vi "LV SciSDK REGISTER FILE SET REGISTER.vi"(8 "error in (no error)":errorcluster, 9 "Register File Handle In":T2, 10 "Register Name":string, 11 "Value":i32) -> (0 "error out":errorcluster, 1 "Register File Handle Out":T2)   [LabVIEW 2021, in "SciSDK_Labview.lvlib"]
uses:
  SciSDK_Labview.lvlib
panel:
  out "NI Error Code":i32
  out "Board Handle Out":T1
  in  "Board Handle In":T1
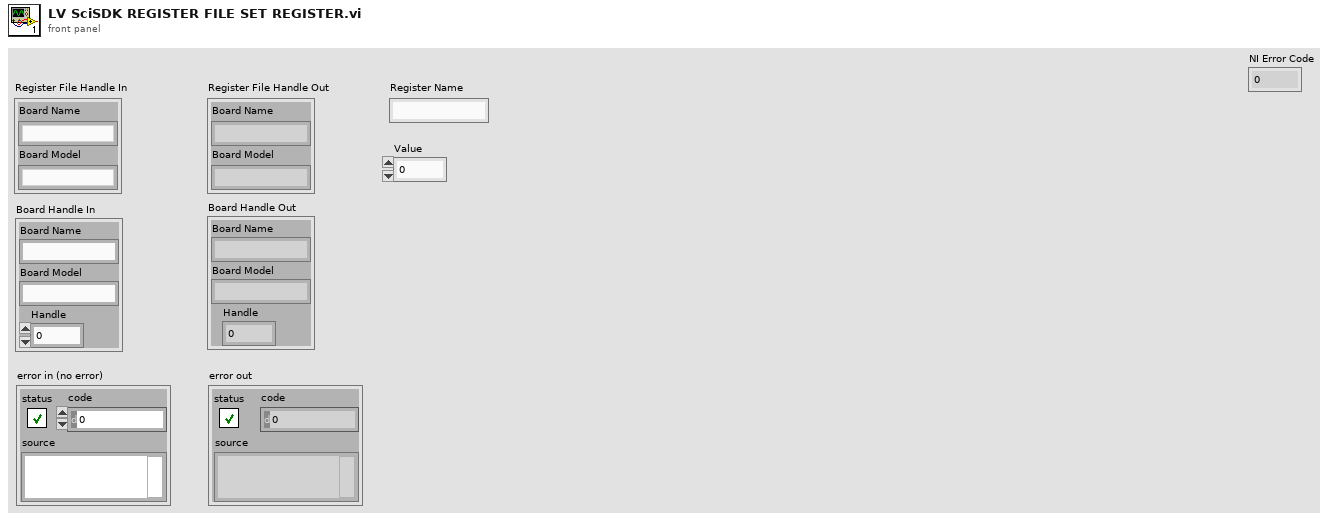
[diagram p1: front panel]
types:
  T1 = cluster{"Board Name":string, "Board Model":string, "Handle":u64}
  T2 = cluster{"Board Name":string, "Board Model":string}
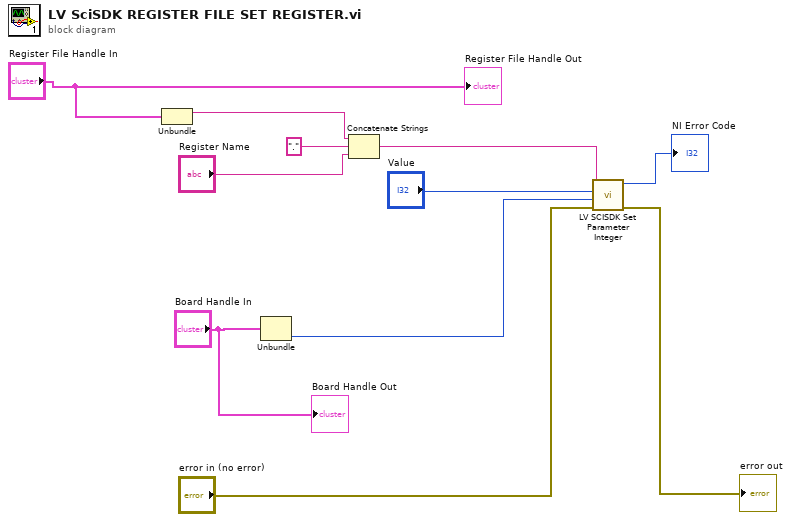
[diagram p0: block diagram]
diagram:
  n1 = Unbundle("Register File Handle In") -> ("Board Name"=w4:string)  [unwired: 1 out]
  n2 = Unbundle("Board Handle In") -> ("Handle"=w2:u64)  [unwired: 2 out]
  n3 = Concatenate Strings(w4, "." ("string"), "Register Name") -> (w8:string)
  n4 = call "LV SCISDK Set Parameter Integer.vi"("error in (no error)"="error in (no error)", "handle"=w2, "value"="Value", "Path"=w8) -> ("error out"=→"error out":errorcluster, "function return"=→"NI Error Code":i32)  [unwired: 5 in, 1 out]
  "Register File Handle Out" <- "Register File Handle In"
  "Board Handle Out" <- "Board Handle In"
